vi "Read Ref.vi"(8 "error in":errorcluster, 11 "Config Data in":refnum<class "Config Data.lvclass">) -> (0 "error out":errorcluster, 2 "config data":T1, 3 "Config Data out":refnum<class "Config Data.lvclass">)   [LabVIEW 2017, in "Config Data.lvclass"]
uses:
  Config Data.lvclass
  <vilib>/Utility/config.llb/Config Data RefNum.ctl
  Config Data.lvclass/Config Data.ctl
  <vilib>/Utility/config.llb/NI_LVConfig.lvlib
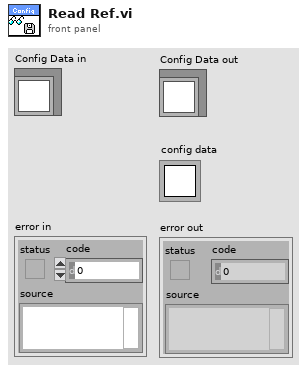
[diagram p1: front panel]
types:
  T1 = typedef "NI_LVConfig.lvlib/Config Data RefNum.ctl" = refnum<k1>
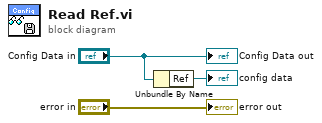
[diagram p0: block diagram]
diagram:
  n1 = Unbundle By Name("Config Data in") -> ("Ref"=→"config data":T1)
  "error out" <- "error in"
  "Config Data out" <- "Config Data in"
